vi "Create Sequence Parameter Assignment.vi"   [LabVIEW 2020, in "NI_VS Sequence Execution Interface.lvlib"]
doc: "Assigns a value to a real-time sequence parameter. The value can be a constant value, data in a file, or a mapping to a channel in a system definition file. Use this VI to create parameter assignment references to use with the Create Sequence Call VI. \n\nWire data to the <B>Channel</B> input to determine the polymorphic instance to use or manually select the instance."
uses:
  <vilib>/NI VeriStand/Execution/SequenceExecutionInterface/NI_VS Sequence Execution Interface.lvlib
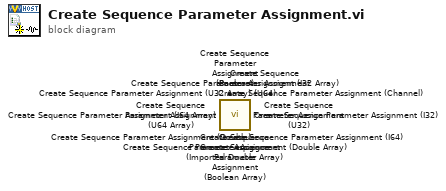
[diagram p0: block diagram]
diagram:
  n1 = call <vilib>:"Create Sequence Parameter Assignment (Imported Double Array).vi"() -> ()  [unwired: 10 in, 2 out]
  n2 = call <vilib>:"Create Sequence Parameter Assignment (U64).vi"() -> ()  [unwired: 10 in, 2 out]
  n3 = call <vilib>:"Create Sequence Parameter Assignment (U64 Array).vi"() -> ()  [unwired: 10 in, 2 out]
  n4 = call <vilib>:"Create Sequence Parameter Assignment (U32).vi"() -> ()  [unwired: 10 in, 2 out]
  n5 = call <vilib>:"Create Sequence Parameter Assignment (U32 Array).vi"() -> ()  [unwired: 10 in, 2 out]
  n6 = call <vilib>:"Create Sequence Parameter Assignment (I64).vi"() -> ()  [unwired: 10 in, 2 out]
  n7 = call <vilib>:"Create Sequence Parameter Assignment (I64 Array).vi"() -> ()  [unwired: 10 in, 2 out]
  n8 = call <vilib>:"Create Sequence Parameter Assignment (I32).vi"() -> ()  [unwired: 10 in, 2 out]
  n9 = call <vilib>:"Create Sequence Parameter Assignment (I32 Array).vi"() -> ()  [unwired: 10 in, 2 out]
  n10 = call <vilib>:"Create Sequence Parameter Assignment (Double).vi"() -> ()  [unwired: 10 in, 2 out]
  n11 = call <vilib>:"Create Sequence Parameter Assignment (Double Array).vi"() -> ()  [unwired: 10 in, 2 out]
  n12 = call <vilib>:"Create Sequence Parameter Assignment (Channel).vi"() -> ()  [unwired: 10 in, 2 out]
  n13 = call <vilib>:"Create Sequence Parameter Assignment (Boolean).vi"() -> ()  [unwired: 10 in, 2 out]
  n14 = call <vilib>:"Create Sequence Parameter Assignment (Boolean Array).vi"() -> ()  [unwired: 10 in, 2 out]
